vi "Digital_Output_32Channels.vi"(1 "States":bool[](array[boolean])=[FALSE, FALSE, FALSE, FALSE, FALSE, FALSE, FALSE, FALSE, FALSE, FALSE, FALSE, FALSE, FALSE, FALSE, FALSE, FALSE, FALSE, FALSE, FALSE, FALSE, FALSE, FALSE, FALSE, FALSE, FALSE, FALSE, FALSE, FALSE, FALSE, FALSE, FALSE, FALSE], 2 "IO":T1={"DO 0"="Mod1/DIO2", "DO 1"="Mod1/DIO2", "DO 2"="Mod1/DIO2", "DO 3"="Mod1/DIO2", "DO 4"="Mod1/DIO2", "DO 5"="Mod1/DIO2", "DO 6"="Mod1/DIO2", "DO 7"="Mod1/DIO2", "DO 8"="Mod1/DIO2", "DO 9"="Mod1/DIO2", "DO 10"="Mod1/DIO2", "DO 11"="Mod1/DIO2", "DO 12"="Mod1/DIO2", "DO 13"="Mod1/DIO2", "DO 14"="Mod1/DIO2", "DO 15"="Mod1/DIO2", "DO 16"="Mod1/DIO2", "DO 17"="Mod1/DIO2", "DO 18"="Mod1/DIO2", "DO 19"="Mod1/DIO2", "DO 20"="Mod1/DIO2", "DO 21"="Mod1/DIO2", "DO 22"="Mod1/DIO2", "DO 23"="Mod1/DIO2", "DO 24"="Mod1/DIO2", "DO 25"="Mod1/DIO2", "DO 26"="Mod1/DIO2", "DO 27"="Mod1/DIO2", "DO 28"="Mod1/DIO2", "DO 29"="Mod1/DIO2", "DO 30"="Mod1/DIO2", "DO 31"="Mod1/DIO2"}) -> ()   [LabVIEW 2015]
uses:
  <vilib>/rvi/eio/common/nirviEmuTemplateMethod_errors.vi
  <vilib>/eio/EIONode/EIONode.xnode
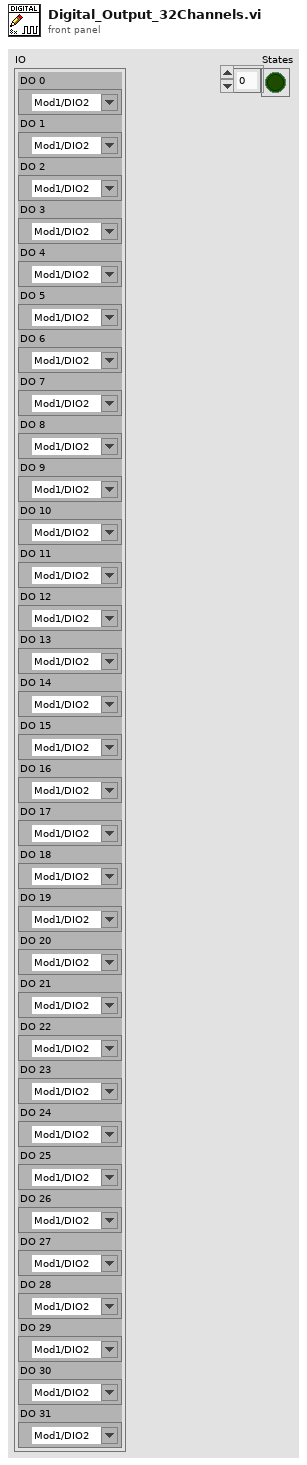
[diagram p1: front panel]
types:
  T1 = cluster{"DO 0":refnum<k21>, "DO 1":refnum<k21>, "DO 2":refnum<k21>, "DO 3":refnum<k21>, "DO 4":refnum<k21>, "DO 5":refnum<k21>, "DO 6":refnum<k21>, "DO 7":refnum<k21>, "DO 8":refnum<k21>, "DO 9":refnum<k21>, "DO 10":refnum<k21>, "DO 11":refnum<k21>, "DO 12":refnum<k21>, "DO 13":refnum<k21>, "DO 14":refnum<k21>, "DO 15":refnum<k21>, "DO 16":refnum<k21>, "DO 17":refnum<k21>, "DO 18":refnum<k21>, "DO 19":refnum<k21>, "DO 20":refnum<k21>, "DO 21":refnum<k21>, "DO 22":refnum<k21>, "DO 23":refnum<k21>, "DO 24":refnum<k21>, "DO 25":refnum<k21>, "DO 26":refnum<k21>, "DO 27":refnum<k21>, "DO 28":refnum<k21>, "DO 29":refnum<k21>, "DO 30":refnum<k21>, "DO 31":refnum<k21>}
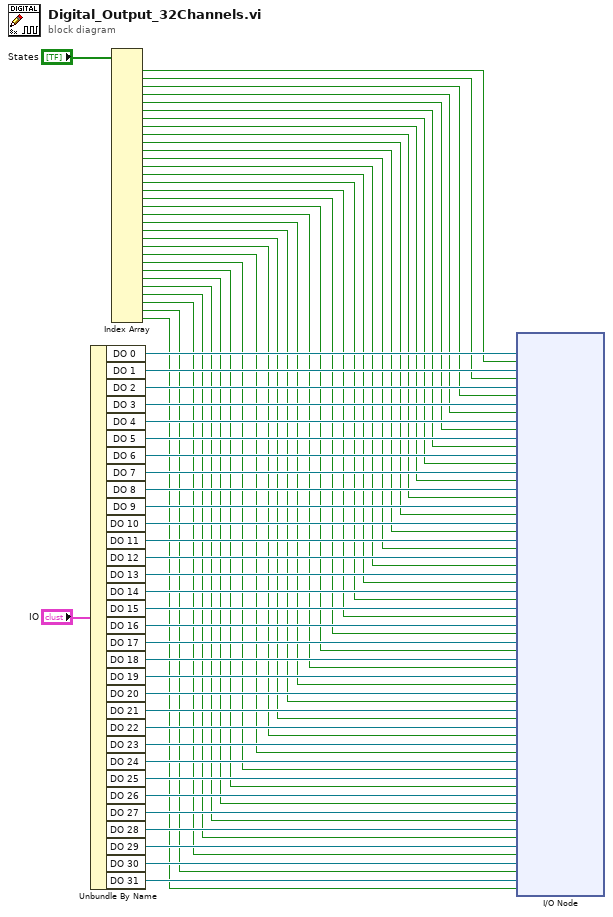
[diagram p0: block diagram]
diagram:
  n1 = Unbundle By Name("IO") -> ("DO 0"=w65:refnum<k21>, "DO 1"=w64:refnum<k21>, "DO 2"=w63:refnum<k21>, "DO 3"=w62:refnum<k21>, "DO 4"=w61:refnum<k21>, "DO 5"=w60:refnum<k21>, "DO 6"=w59:refnum<k21>, "DO 7"=w58:refnum<k21>, "DO 8"=w48:refnum<k21>, "DO 9"=w47:refnum<k21>, "DO 10"=w46:refnum<k21>, "DO 11"=w45:refnum<k21>, "DO 12"=w44:refnum<k21>, "DO 13"=w43:refnum<k21>, "DO 14"=w42:refnum<k21>, "DO 15"=w41:refnum<k21>, "DO 16"=w40:refnum<k21>, "DO 17"=w39:refnum<k21>, "DO 18"=w38:refnum<k21>, "DO 19"=w37:refnum<k21>, "DO 20"=w36:refnum<k21>, "DO 21"=w35:refnum<k21>, "DO 22"=w34:refnum<k21>, "DO 23"=w33:refnum<k21>, "DO 24"=w32:refnum<k21>, "DO 25"=w31:refnum<k21>, "DO 26"=w30:refnum<k21>, "DO 27"=w29:refnum<k21>, "DO 28"=w28:refnum<k21>, "DO 29"=w27:refnum<k21>, "DO 30"=w26:refnum<k21>, "DO 31"=w25:refnum<k21>)
  n2 = Index Array(array="States") -> (element #1=w56:bool, element #2=w55:bool, element #3=w54:bool, element #4=w53:bool, element #5=w52:bool, element #6=w51:bool, element #7=w50:bool, element #8=w49:bool, element #9=w24:bool, element #10=w23:bool, element #11=w22:bool, element #12=w21:bool, element #13=w20:bool, element #14=w19:bool, element #15=w18:bool, element #16=w17:bool, element #17=w16:bool, element #18=w15:bool, element #19=w14:bool, element #20=w13:bool, element #21=w12:bool, element #22=w11:bool, element #23=w10:bool, element #24=w9:bool, element #25=w8:bool, element #26=w7:bool, element #27=w6:bool, element #28=w5:bool, element #29=w4:bool, element #30=w3:bool, element #31=w2:bool, element #32=w1:bool)  [unwired: 32 in]
  n3 = xnode "I/O Node"("I/O Item"=w56, "FPGA I/O In"=w65, "I/O Item"=w55, "FPGA I/O In"=w64, "I/O Item"=w54, "FPGA I/O In"=w63, "I/O Item"=w53, "FPGA I/O In"=w62, "I/O Item"=w52, "FPGA I/O In"=w61, "I/O Item"=w51, "FPGA I/O In"=w60, "I/O Item"=w50, "FPGA I/O In"=w59, "I/O Item"=w49, "FPGA I/O In"=w58, "I/O Item"=w24, "FPGA I/O In"=w48, "I/O Item"=w23, "FPGA I/O In"=w47, "I/O Item"=w22, "FPGA I/O In"=w46, "I/O Item"=w21, "FPGA I/O In"=w45, "I/O Item"=w20, "FPGA I/O In"=w44, "I/O Item"=w19, "FPGA I/O In"=w43, "I/O Item"=w18, "FPGA I/O In"=w42, "I/O Item"=w17, "FPGA I/O In"=w41, "I/O Item"=w16, "FPGA I/O In"=w40, "I/O Item"=w15, "FPGA I/O In"=w39, "I/O Item"=w14, "FPGA I/O In"=w38, "I/O Item"=w13, "FPGA I/O In"=w37, "I/O Item"=w12, "FPGA I/O In"=w36, "I/O Item"=w11, "FPGA I/O In"=w35, "I/O Item"=w10, "FPGA I/O In"=w34, "I/O Item"=w9, "FPGA I/O In"=w33, "I/O Item"=w8, "FPGA I/O In"=w32, "I/O Item"=w7, "FPGA I/O In"=w31, "I/O Item"=w6, "FPGA I/O In"=w30, "I/O Item"=w5, "FPGA I/O In"=w29, "I/O Item"=w4, "FPGA I/O In"=w28, "I/O Item"=w3, "FPGA I/O In"=w27, "I/O Item"=w2, "FPGA I/O In"=w26, "I/O Item"=w1, "FPGA I/O In"=w25) -> ()  [unwired: 32 out]
